vi "lua_gc.vi"(4 "stepmul (majormul)":i32, 6 "stepsize (minormul)":i32, 8 "error in (no error)":errorcluster, 9 "pause?":bool, 10 "what":T1, 11 "lua_state_p":u64) -> (0 "error out":errorcluster, 2 "result":i32, 3 "lua_state_p out":u64)   [LabVIEW 2020, in "lua.dll.lvlib"]
doc: "Controls the garbage collector.\n\nThis function performs several tasks, according to the value of the parameter what. For options that need extra arguments, they are listed after the option.\n\nLUA_GCCOLLECT: Performs a full garbage-collection cycle.\nLUA_GCSTOP: Stops the garbage collector.\nLUA_GCRESTART: Restarts the garbage collector.\nLUA_GCCOUNT: Returns the current amount of memory (in Kbytes) in use by Lua.\nLUA_GCCOUNTB: Returns the remainder of dividing the current amount of bytes of memory in use by Lua by 1024.\nLUA_GCSTEP (int stepsize): Performs an incremental step of garbage collection, corresponding to the allocation of stepsize Kbytes.\nLUA_GCISRUNNING: Returns a boolean that tells whether the collector is running (i.e., not stopped).\nLUA_GCINC (int pause, int stepmul, stepsize): Changes the collector to incremental mode with the given parameters (see §2.5.1). Returns the previous mode (LUA_GCGEN or LUA_GCINC).\nLUA_GCGEN (int minormul, int majormul): Changes the collector to generational mode with the given parameters (see §2.5.2). Returns the previous mode (LUA_GCGEN or LUA_GCINC).\nFor more details about these options, see collectgarbage."
uses:
  lua.dll.lvlib
  lua54.dll
  types/LUA_GC.ctl
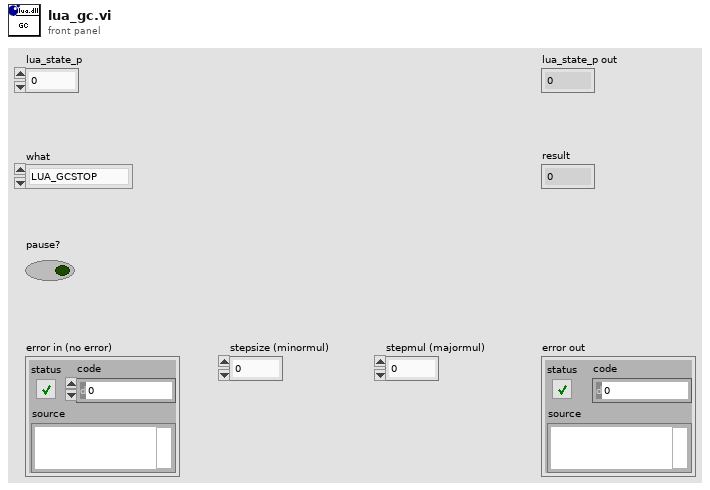
[diagram p1: front panel]
types:
  T1 = typedef "lua.dll.lvlib/LUA_GC.ctl" = enum32{"LUA_GCSTOP", "LUA_GCRESTART", "LUA_GCCOLLECT", "LUA_GCCOUNT", "LUA_GCCOUNTB", "LUA_GCSTEP", "LUA_GCSETPAUSE", "LUA_GCSETSTEPMUL", "LUA_GCSETMAJORINC", "LUA_GCISRUNNING", "LUA_GCGEN", "LUA_GCINC"}
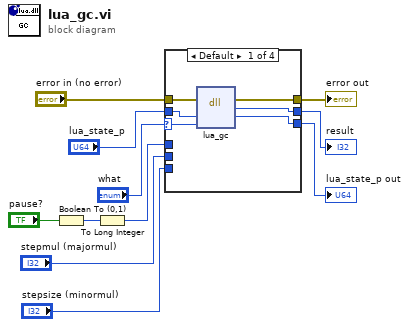
[diagram p0: block diagram]
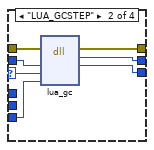
[diagram p2: hidden frame]
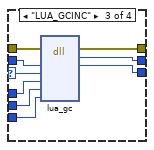
[diagram p3: hidden frame]
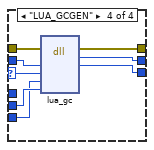
[diagram p4: hidden frame]
diagram:
  n1 = Boolean To (0,1)(Boolean="pause?") -> (0, 1=w4:i16)
  n2 = To Long Integer(number=w4) -> (32bit integer=w1:i32)
  n3 = case shown="Default" "what" {
    selector: "what" -> [w12 w19 w28 w36]
    tunnel: "error in (no error)" -> [w17 w24 w33 w41]
    tunnel: [w16 w23 w32 w40] -> w10
    tunnel: "lua_state_p" -> [w15 w22 w31 w39]
    tunnel: [w14 w21 w30 w38] -> w8
    tunnel: [w13 w20 w29 w37] -> w7
    tunnel: "stepsize (minormul)" -> [_ w18 w26 w34]
    tunnel: w1 -> [_ _ w27 _]
    tunnel: "stepmul (majormul)" -> [_ _ w25 w35]
    frame Default {
      n4 = dll-call lib="C:/Users/Nicholas Folse/Documents/workspace/github-tauterra.llc/Lua for LabVIEW/lib/lua.dll/lua54**.*" fn="lua_gc"(error in=w17, "lua_state_p"=w15, "what"=w12) -> (error out=w16:errorcluster, "type"=w13:i32, "lua_state_p"=w14:u64)  [unwired: 3 in, 1 out]
    }
    frame "LUA_GCSTEP" {
      n5 = dll-call lib="C:/Users/Nicholas Folse/Documents/workspace/github-tauterra.llc/Lua for LabVIEW/lib/lua.dll/lua54**.*" fn="lua_gc"(error in=w24, "lua_state_p"=w22, "what"=w19, "stepsize"=w18) -> (error out=w23:errorcluster, "type"=w20:i32, "lua_state_p"=w21:u64)  [unwired: 4 in, 1 out]
    }
    frame "LUA_GCINC" {
      n6 = dll-call lib="C:/Users/Nicholas Folse/Documents/workspace/github-tauterra.llc/Lua for LabVIEW/lib/lua.dll/lua54**.*" fn="lua_gc"(error in=w33, "lua_state_p"=w31, "what"=w28, "pause"=w27, "stepmul"=w25, "stepsize"=w26) -> (error out=w32:errorcluster, "type"=w29:i32, "lua_state_p"=w30:u64)  [unwired: 6 in, 1 out]
    }
    frame "LUA_GCGEN" {
      n7 = dll-call lib="C:/Users/Nicholas Folse/Documents/workspace/github-tauterra.llc/Lua for LabVIEW/lib/lua.dll/lua54**.*" fn="lua_gc"(error in=w41, "lua_state_p"=w39, "what"=w36, "minormul"=w34, "majormul"=w35) -> (error out=w40:errorcluster, "type"=w37:i32, "lua_state_p"=w38:u64)  [unwired: 5 in, 1 out]
    }
  }
  "error out" <- w10
  "lua_state_p out" <- w8
  "result" <- w7
